vi "Write Experiment Parameter Values.vi"(8 "error in (no error)":errorcluster, 10 "Experiment Parameter Values":T1(array[cluster]), 11 "TrialBasedExperiment in":refnum<class "TrialBasedExperiment.lvclass">) -> (0 "error out":errorcluster, 3 "TrialBasedExperiment out":refnum<class "TrialBasedExperiment.lvclass">)   [LabVIEW 2010]
uses:
  TrialBasedExperiment.lvclass
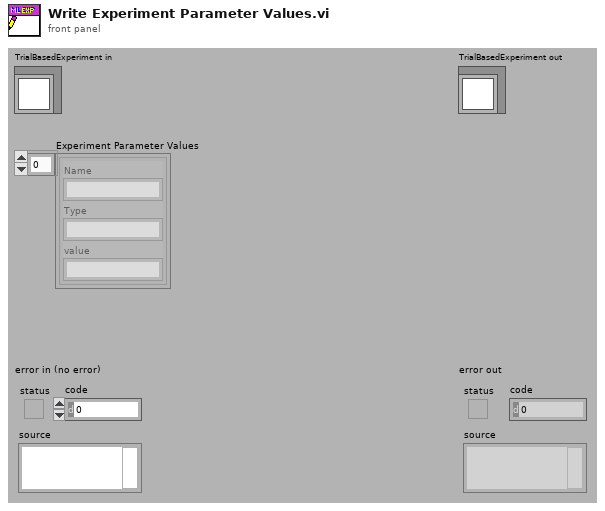
[diagram p1: front panel]
types:
  T1 = cluster{"Name":string, "Type":string, "value":string}[]
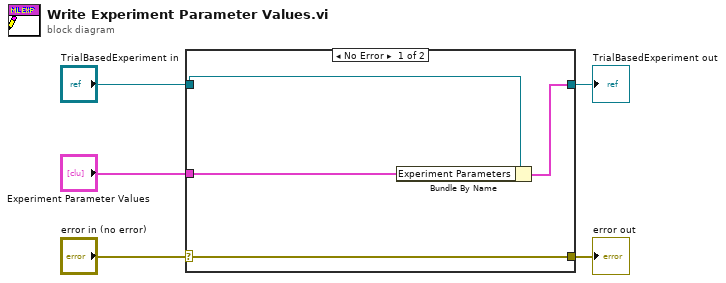
[diagram p0: block diagram]
diagram:
  n1 = case shown="No Error" "error in (no error)" {
    selector: "error in (no error)" -> [w9 w10]
    tunnel: [w9 w10] -> w4
    tunnel: [w7 w11] -> w2
    tunnel: "TrialBasedExperiment in" -> [w8 w11]
    tunnel: "Experiment Parameter Values" -> [w6 _]
    frame No Error {
      n2 = Bundle By Name(cluster=w8, "Experiment Parameters"=w6) -> (w7:cluster{})
    }
    frame Error {
    }
  }
  "error out" <- w4
  "TrialBasedExperiment out" <- w2
